vi "FuelFlap.vi"(11 "Fuel Flap":bool) -> ()   [LabVIEW 2016]
uses:
  <vilib>/Rock Robotics/WPI/Solenoid/Deprecated/WPI_SolenoidSetBool.vi
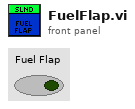
[diagram p1: front panel]
types:
  T1 = typedef "WPI_SolenoidDevRef.ctl" = cluster{"DevStatus":errorcluster, "Pneumatics Control Module":u8, "Forward Solenoid Channel":T2, "Reverse Solenoid Channel":T2}
  T2 = typedef "WPI_SolenoidChannel.ctl" = enum8{"Solenoid 0", "Solenoid 1", "Solenoid 2", "Solenoid 3", "Solenoid 4", "Solenoid 5", "Solenoid 6", "Solenoid 7", "Invalid"}
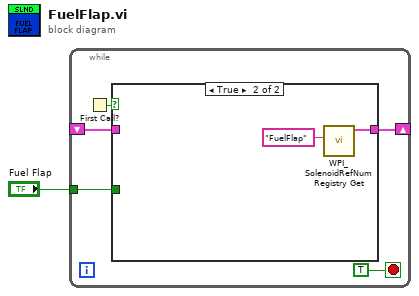
[diagram p0: block diagram]
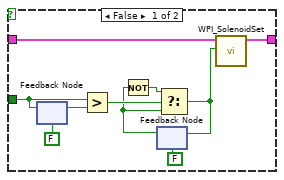
[diagram p2: hidden frame]
diagram:
  n1 = while {
    shift-right: [w5] -> _
    shift-left: _ -> [w4]
    tunnel: "Fuel Flap" -> [w2]
    stop <- TRUE stop-if-true
    n2 = First Call?() -> (First Call?: T/F=w6:bool)
    n3 = case shown="True" w6 {
      tunnel: [w16 w18] -> w5
      tunnel: w4 -> [w15 _]
      tunnel: w2 -> [w7 _]
      frame False {
        n4 = feedback-in #1(w7) -> ()
        n5 = feedback #1(FALSE ("Fuel Flap")) -> (w13:bool)
        n6 = Greater?(x=w7, y=w13) -> (0:w12:bool)
        n7 = feedback #2(FALSE) -> (w10:bool)
        n8 = Not(x=w10) -> (.not. x?=w11:bool)
        n9 = Select(t=w11, s=w12, f=w10) -> (s? t:f=w9:bool)
        n10 = feedback-in #2(w9) -> ()
        n11 = call-poly <vilib>:"WPI_SolenoidSet.vi"("Value"=w9, "SolenoidDevRef"=w15) -> ("SolenoidDevRef"=w16:T1)  [unwired: 8 in, 1 out]
      }
      frame True {
        n12 = call <vilib>:"WPI_SolenoidRefNum Registry Get.vi"("refnum name"="FuelFlap") -> ("SolenoidDevRef"=w18:T1)  [unwired: 9 in, 1 out]
      }
    }
  }
